vi "Run Process.vi"(8 "error in (no error)":errorcluster, 9 "Processes":cluster{"VI":refnum<vi>, "Parameters":variant}[](array[cluster]), 11 "Async in":refnum<class "VS Inline Async API.lvclass">) -> (0 "error out":errorcluster, 3 "Async out":refnum<class "VS Inline Async API.lvclass">)   [LabVIEW 2015, in "VS Inline Async API.lvlib" / "VS Inline Async API.lvclass"]
uses:
  VS Inline Async API.lvclass
  VS Inline Async API.lvclass/VS Inline Async API.ctl
  Process/Process.lvclass
  Process/Process.lvclass/Process.ctl
  Process/Data Member Access/Write Name.vi
  Process/Data Member Access/Write Process.Stop.vi
  Process/Data Member Access/Write Process.Trigger.vi
  Process/Data Member Access/Write Data Access.vi
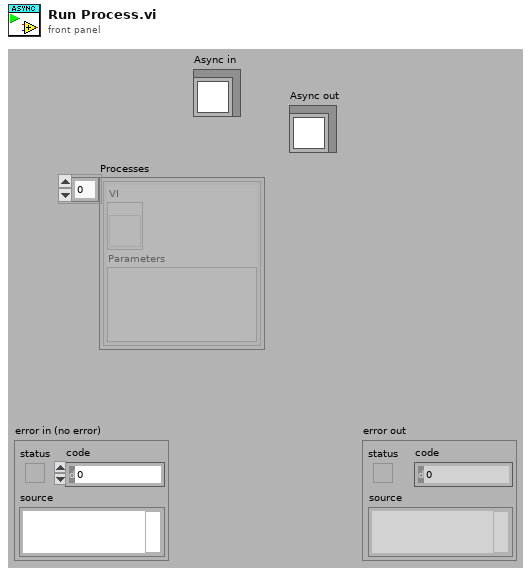
[diagram p1: front panel]
types:
  T1 = cluster{"read mode":enum16{"polling", "blocking"}, "write mode":enum16{"polling", "blocking"}}
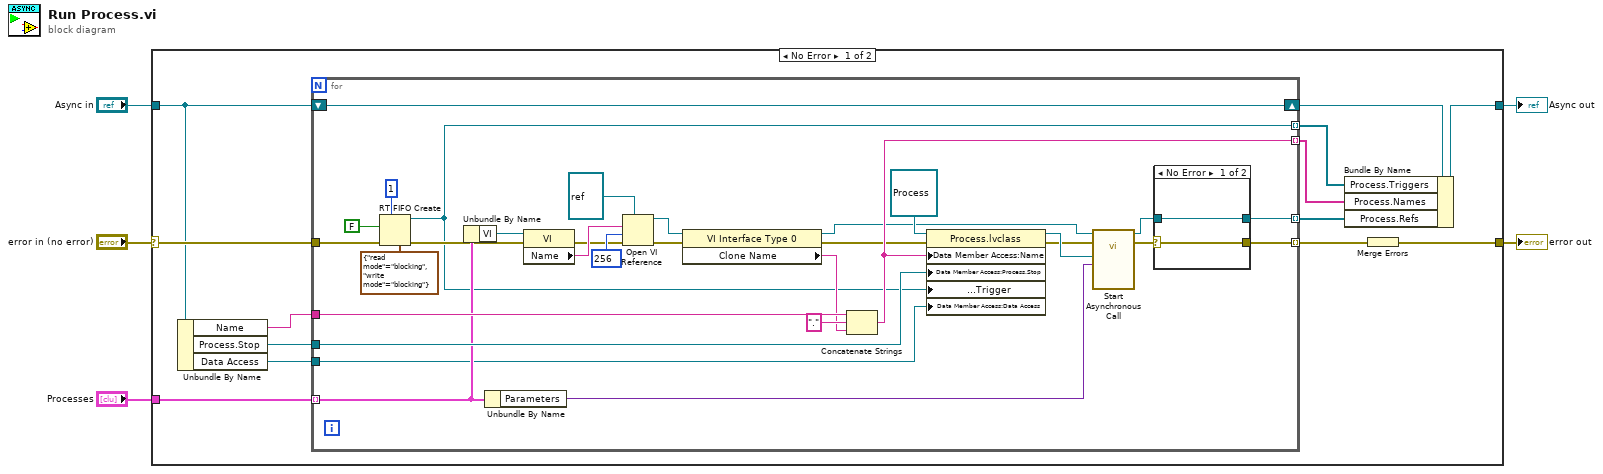
[diagram p0: block diagram]
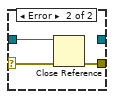
[diagram p2: hidden frame]
diagram:
  n1 = case shown="No Error" "error in (no error)" {
    selector: "error in (no error)" -> [w17 w56]
    tunnel: [w15 w56] -> w5
    tunnel: "Processes" -> [w16 _]
    tunnel: "Async in" -> [w11 w55]
    tunnel: [w12 w55] -> w1
    frame No Error {
      n2 = Unbundle By Name(w11) -> ("Name"=w10:string, "Process.Stop"=w9:refnum<data-value>, "Data Access"=w7:refnum<class "Data Access Engine.lvclass">)
      n3 = for {
        tunnel: [w49] -> w18 mode=indexing
        tunnel: [w48] -> w14 mode=indexing
        tunnel: w17 -> [w24]
        tunnel: w16 -> [w35] mode=indexing
        shift-right: [w44] -> w13
        shift-left: w11 -> [w44]
        tunnel: w10 -> [w43]
        tunnel: w9 -> [w39]
        tunnel: [w37] -> w8 mode=indexing
        tunnel: w7 -> [w33]
        tunnel: [w19] -> w6 mode=indexing
        n4 = RT FIFO Create(1:FALSE, 3:w24, 4:u32 1 ("size (10)"), 7:T1 {"read mode"=enum."blocking", "write mode"=enum."blocking"} ("r/w modes (polling,polling)")) -> (8:w19:refnum<k33>, 11:w23:errorcluster)  [unwired: 4 in, 1 out]
        n5 = Unbundle By Name(w35) -> ("VI"=w36:refnum<vi>)
        n6 = Unbundle By Name(w35) -> ("Parameters"=w34:variant)
        n7 = property class="VI"(reference=w36, error in=w23) -> (error out=w28:errorcluster, "Name"=w42:string)  [unwired: 1 out]
        n8 = Open VI Reference(type specifier VI Refnum (for type only)=refnum<vi> refnum, vi path=w42, options=256, error in (no error)=w28) -> (vi reference=w31:refnum<vi>, error out=w32:errorcluster)  [unwired: 2 out]
        n9 = property class="VI Interface Type 0"(reference=w31, error in=w32) -> (reference out=w30:refnum<vi>, error out=w29:errorcluster, "Clone Name"=w27:string)
        n10 = Concatenate Strings(w43, "." ("string"), w27) -> (w37:string)
        n11 = property class="Process.lvclass"(reference=refnum<class "Process.lvclass"> refnum ("VS Inline Async API.lvlib:Process.lvclass"), error in=w29, "Data Member Access:Name"=w37, "Data Member Access:Process.Stop"=w39, "Data Member Access:Process.Trigger"=w19, "Data Member Access:Data Access"=w33) -> (reference out=w38:refnum<class "Process.lvclass">, error out=w26:errorcluster)
        n12 = call-by-ref "Start Asynchronous Call"(reference=w30, error in=w26, "Parameters"=w34, "Process"=w38) -> (reference out=w46:refnum<vi>, error out=w47:errorcluster)  [unwired: 10 in]
        n13 = case shown="No Error" w47 {
          selector: w47 -> [w51 w54]
          tunnel: w46 -> [w50 w53]
          tunnel: [w51 w52] -> w49
          tunnel: [w50 _] -> w48
          frame No Error {
          }
          frame Error {
            n14 = Close Reference(reference=w53, error in (no error)=w54) -> (error out=w52:errorcluster)
          }
        }
      }
      n15 = Bundle By Name(cluster=w13, "Process.Triggers"=w6, "Process.Names"=w8, "Process.Refs"=w14) -> (w12:refnum<class "VS Inline Async API.lvclass">)
      n16 = Merge Errors(w18) -> (w15:errorcluster)
    }
    frame Error {
    }
  }
  "error out" <- w5
  "Async out" <- w1
